vi "Analyze.vi"(0 "Analyze Timer in":refnum<class "Analyze Timer.lvclass">, 1 "Create Overlay?":bool, 5 "Image in":T1, 7 "Parameters":variant, 9 "Results in":variant, 11 "error in (no error)":errorcluster) -> (4 "Analyze Timer out":refnum<class "Analyze Timer.lvclass">, 6 "Image out":T1, 8 "Parameters out":variant, 10 "Results":variant, 15 "error out":errorcluster)   [LabVIEW 2020, in "Analyze.lvlib" / "Analyze Timer.lvclass"]
uses:
  Analyze Timer.lvclass
  <vilib>/vision/Image Controls.llb/IMAQ Image.ctl
  Analyze Timer.lvclass/Analyze Timer.ctl
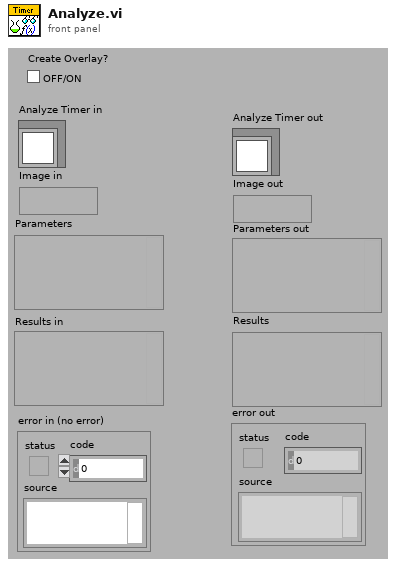
[diagram p1: front panel]
types:
  T1 = typedef "IMAQ Image.ctl" = refnum<image>
  T2 = enum32{"Invalid", "Standard", "Closed", "Hidden", "Minimized", "Maximized"}
  T3 = typedef "LVRectTypeDef.ctl" = cluster{"left":i16, "top":i16, "right":i16, "bottom":i16}
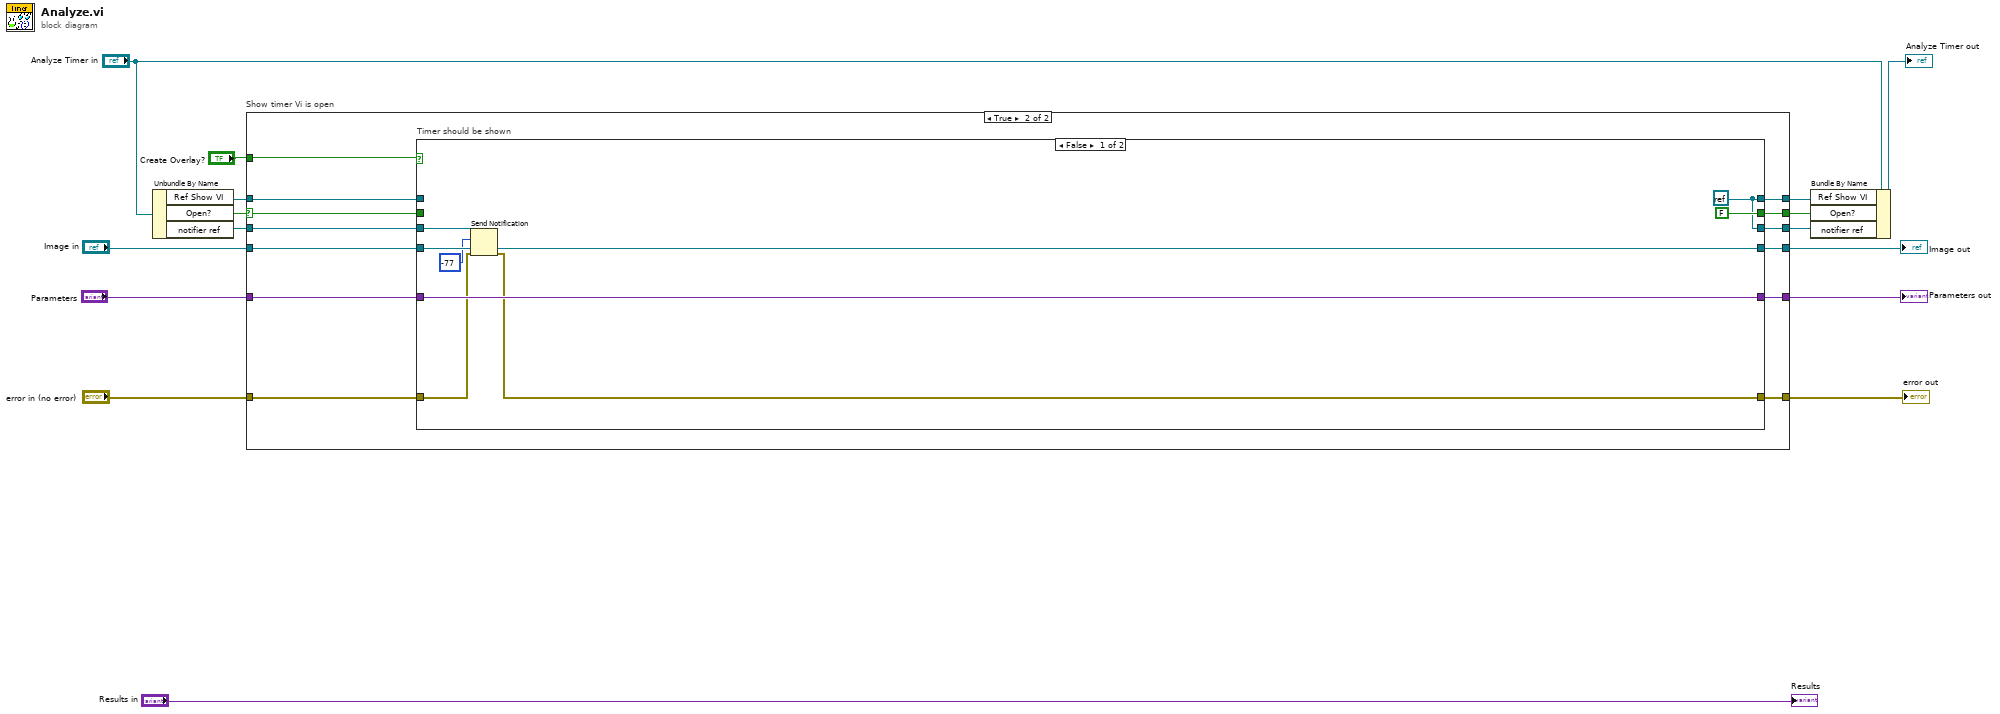
[diagram p0: block diagram]
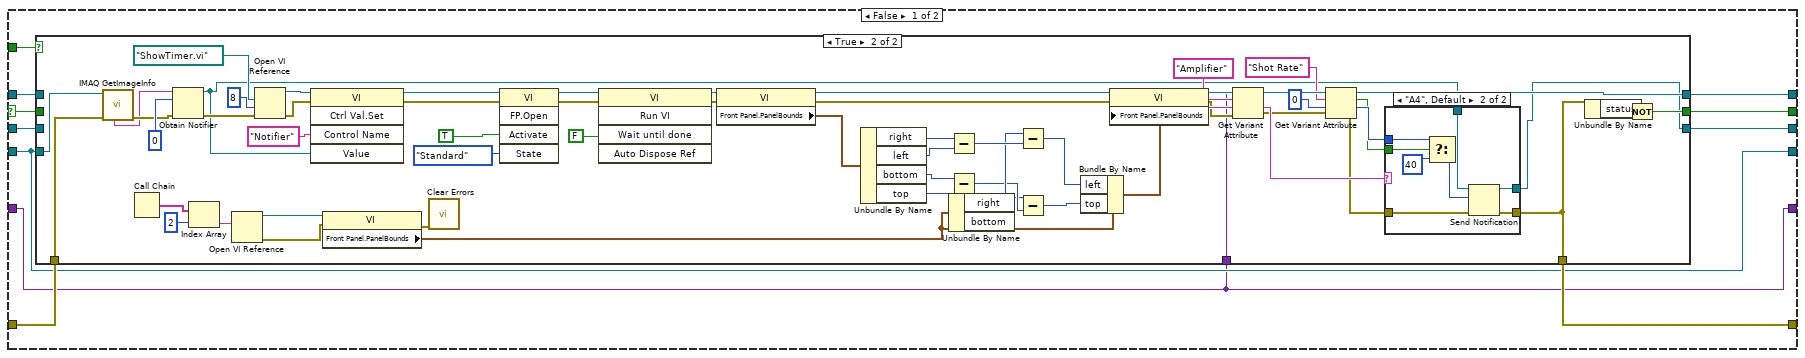
[diagram p2: hidden frame]
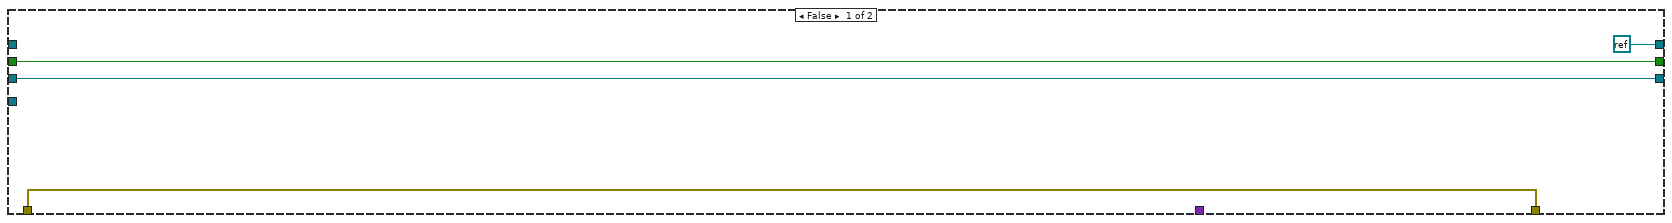
[diagram p3: hidden frame]
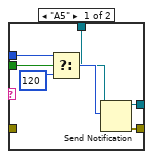
[diagram p4: hidden frame]
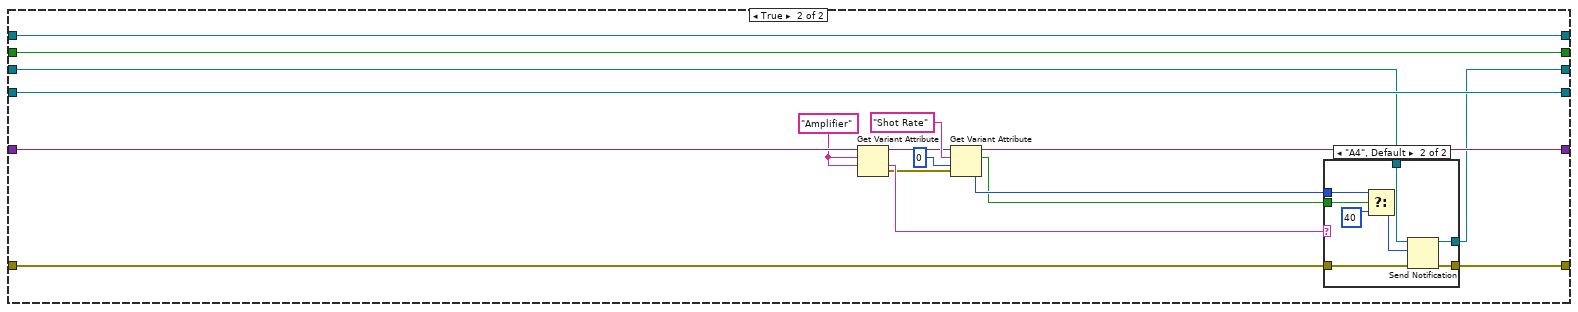
[diagram p5: hidden frame]
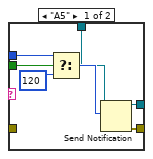
[diagram p6: hidden frame]
diagram:
  n1 = Unbundle By Name("Analyze Timer in") -> ("Ref Show VI"=w10:refnum<vi>, "Open?"=w11:bool, "notifier ref"=w1:refnum<notifier>)
  n2 = case "Show timer Vi is open" shown="True" w11 {
    selector: w11 -> [w23 w108]
    tunnel: [w27 w109] -> w13
    tunnel: "Create Overlay?" -> [w26 w117]
    tunnel: w10 -> [w25 w116]
    tunnel: [w24 w115] -> w9
    tunnel: "Image in" -> [w19 w114]
    tunnel: "Parameters" -> [w17 w113]
    tunnel: "error in (no error)" -> [w22 w112]
    tunnel: [w19 w111] -> w5
    tunnel: [w17 w110] -> w4
    tunnel: [w21 w107] -> w3
    tunnel: [w20 w106] -> w2
    tunnel: w1 -> [w18 w105]
    frame False {
      n3 = case shown="True" w26 {
        tunnel: [w30 w83] -> w27
        tunnel: w25 -> [_ _]
        tunnel: [refnum<k0> refnum w48] -> w24
        tunnel: w23 -> [w30 _]
        tunnel: w22 -> [w29 w79]
        tunnel: [w29 w35] -> w21
        tunnel: [w28 w33] -> w20
        tunnel: w19 -> [_ w78]
        tunnel: w18 -> [w28 _]
        tunnel: w17 -> [_ w32]
        frame False {
        }
        frame True {
          w39 = "Amplifier" ("name")
          n4 = call "IMAQ GetImageInfo"("error in (no error)"=w79, "Image"=w78) -> ("error out"=w77:errorcluster, "Image Name"=w75:string)  [unwired: 2 in, 6 out]
          n5 = Call Chain() -> (call chain=w68:string[])
          n6 = Obtain Notifier(name (unnamed)=w75, notification data type=0, error in (no error)=w77) -> (notifier out=w34:refnum<notifier>, error out=w76:errorcluster)  [unwired: 1 in, 1 out]
          n7 = Index Array(array=w68, index=2) -> (element=w69:string)
          n8 = Open VI Reference(vi path=w69) -> (vi reference=w66:refnum<vi>, error out=w65:errorcluster)  [unwired: 5 in]
          n9 = Open VI Reference(vi path=path "ShowTimer.vi", options=8, error in (no error)=w76) -> (vi reference=w73:refnum<vi>, error out=w71:errorcluster)  [unwired: 3 in]
          n10 = invoke class="VI" method="Ctrl Val.Set"(reference=w73, error in=w71, "Control Name"="Notifier", "Value"=w34) -> (reference out=w72:refnum<vi>, error out=w70:errorcluster)  [unwired: 1 in, 3 out]
          n11 = property class="VI"(reference=w66, error in=w65) -> (error out=w46:errorcluster, "Front Panel.PanelBounds"=w57:T3)  [unwired: 1 out]
          n12 = call <vilib>:"Clear Errors.vi"("error in (no error)"=w46) -> ()  [unwired: 5 in, 2 out]
          n13 = invoke class="VI" method="FP.Open"(reference=w72, error in=w70, "Activate"=TRUE ("Activate?"), "State"=T2."Standard") -> (reference out=w88:refnum<vi>, error out=w87:errorcluster)  [unwired: 1 in, 3 out]
          n14 = invoke class="VI" method="Run VI"(reference=w88, error in=w87, "Wait until done"=FALSE ("Wait Until Done")) -> (reference out=w59:refnum<vi>, error out=w58:errorcluster)  [unwired: 2 in, 3 out]
          n15 = property class="VI"(reference=w59, error in=w58) -> (reference out=w47:refnum<vi>, error out=w49:errorcluster, "Front Panel.PanelBounds"=w64:T3)
          n16 = Unbundle By Name(w64) -> ("right"=w63:i16, "left"=w62:i16, "bottom"=w61:i16, "top"=w60:i16)
          n17 = Subtract(x=w63, y=w62) -> (x-y=w55:i16)
          n18 = Subtract(x=w61, y=w60) -> (x-y=w52:i16)
          n19 = Unbundle By Name(w57) -> ("right"=w54:i16, "bottom"=w51:i16)
          n20 = Subtract(x=w54, y=w55) -> (x-y=w53:i16)
          n21 = Subtract(x=w51, y=w52) -> (x-y=w50:i16)
          n22 = Bundle By Name(cluster=w57, "left"=w53, "top"=w50) -> (w56:T3)
          n23 = property class="VI"(reference=w47, error in=w49, "Front Panel.PanelBounds"=w56) -> (reference out=w48:refnum<vi>, error out=w36:errorcluster)
          n24 = Get Variant Attribute(Variant=w32, name=w39, default value (empty Variant)=w39, error in=w36) -> (duplicate Variant=w41:variant, value=w40:string, error out=w38:errorcluster)  [unwired: 1 out]
          n25 = Get Variant Attribute(Variant=w41, name="Shot Rate", default value (empty Variant)=0, error in=w38) -> (found=w44:bool, value=w45:i32, error out=w37:errorcluster)  [unwired: 1 out]
          n26 = case shown="\"A4\", Default" w40 {
            tunnel: w44 -> [w95 w103]
            tunnel: w45 -> [w94 w102]
            tunnel: [w92 w100] -> w33
            tunnel: [w91 w99] -> w35
            tunnel: w34 -> [w90 w98]
            tunnel: w37 -> [_ w97]
            frame "A5" {
              n27 = Select(t=w94, s=w95, f=120 ("notification")) -> (s? t:f=w93:i32)
              n28 = Send Notification(notification=w93, notifier=w90) -> (notifier out=w92:refnum<notifier>, error out=w91:errorcluster)  [unwired: 1 in]
            }
            frame "A4", Default {
              n29 = Select(t=w102, s=w103, f=40 ("notification")) -> (s? t:f=w101:i32)
              n30 = Send Notification(notification=w101, notifier=w98, error in (no error)=w97) -> (notifier out=w100:refnum<notifier>, error out=w99:errorcluster)
            }
          }
          n31 = Unbundle By Name(w35) -> ("status"=w84:bool)
          n32 = Not(x=w84) -> (.not. x?=w83:bool)
        }
      }
    }
    frame True {
      n33 = case "Timer should be shown" shown="False" w117 {
        tunnel: w116 -> [_ w132]
        tunnel: [w122 w132] -> w115
        tunnel: w114 -> [w125 w134]
        tunnel: w113 -> [w124 w136]
        tunnel: w112 -> [w119 w127]
        tunnel: [w125 w134] -> w111
        tunnel: [w124 w133] -> w110
        tunnel: [FALSE w131] -> w109
        tunnel: w108 -> [_ w131]
        tunnel: [w118 w126] -> w107
        tunnel: [w122 w128] -> w106
        tunnel: w105 -> [w121 w129]
        frame False {
          w122 = refnum<k0> refnum
          n34 = Send Notification(notification=-77, notifier=w121, error in (no error)=w119) -> (error out=w118:errorcluster)  [unwired: 1 out]
        }
        frame True {
          w135 = "Amplifier" ("name")
          n35 = Get Variant Attribute(Variant=w136, name=w135, default value (empty Variant)=w135) -> (duplicate Variant=w138:variant, value=w137:string, error out=w130:errorcluster)  [unwired: 1 in, 1 out]
          n36 = Get Variant Attribute(Variant=w138, name="Shot Rate", default value (empty Variant)=0, error in=w130) -> (duplicate Variant=w133:variant, found=w141:bool, value=w142:i32)  [unwired: 1 out]
          n37 = case shown="\"A4\", Default" w137 {
            tunnel: w141 -> [w148 w156]
            tunnel: w142 -> [w147 w155]
            tunnel: [w145 w153] -> w128
            tunnel: [w144 w152] -> w126
            tunnel: w129 -> [w143 w151]
            tunnel: w127 -> [_ w150]
            frame "A5" {
              n38 = Select(t=w147, s=w148, f=120 ("notification")) -> (s? t:f=w146:i32)
              n39 = Send Notification(notification=w146, notifier=w143) -> (notifier out=w145:refnum<notifier>, error out=w144:errorcluster)  [unwired: 1 in]
            }
            frame "A4", Default {
              n40 = Select(t=w155, s=w156, f=40 ("notification")) -> (s? t:f=w154:i32)
              n41 = Send Notification(notification=w154, notifier=w151, error in (no error)=w150) -> (notifier out=w153:refnum<notifier>, error out=w152:errorcluster)
            }
          }
        }
      }
    }
  }
  "error out" <- w3
  "Parameters out" <- w4
  "Image out" <- w5
  n42 = Bundle By Name(cluster="Analyze Timer in", "Ref Show VI"=w9, "Open?"=w13, "notifier ref"=w2) -> (→"Analyze Timer out":refnum<class "Analyze Timer.lvclass">)
  "Results" <- "Results in"
